vi "CountPulses60.vi"(9 "60bit input":bool[](array[boolean])=[FALSE, FALSE, FALSE, FALSE, FALSE, FALSE, FALSE, FALSE, FALSE, FALSE, FALSE, FALSE, FALSE, FALSE, FALSE, FALSE, FALSE, FALSE, FALSE, FALSE, FALSE, FALSE, FALSE, FALSE, FALSE, FALSE, FALSE, FALSE, FALSE, FALSE, FALSE, FALSE, FALSE, FALSE, FALSE, FALSE, FALSE, FALSE, FALSE, FALSE, FALSE, FALSE, FALSE, FALSE, FALSE, FALSE, FALSE, FALSE, FALSE, FALSE, FALSE, FALSE, FALSE, FALSE, FALSE, FALSE, FALSE, FALSE, FALSE, FALSE], 10 "Previous pulse count":u16, 11 "Last sample":bool) -> (2 "New pulse count":u16, 3 "New last sample":bool)   [LabVIEW 2012]
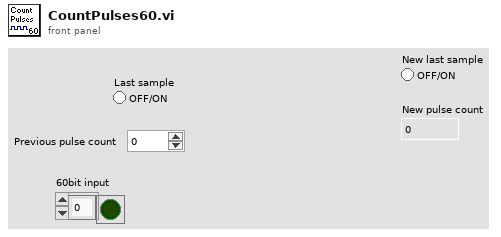
[diagram p1: front panel]
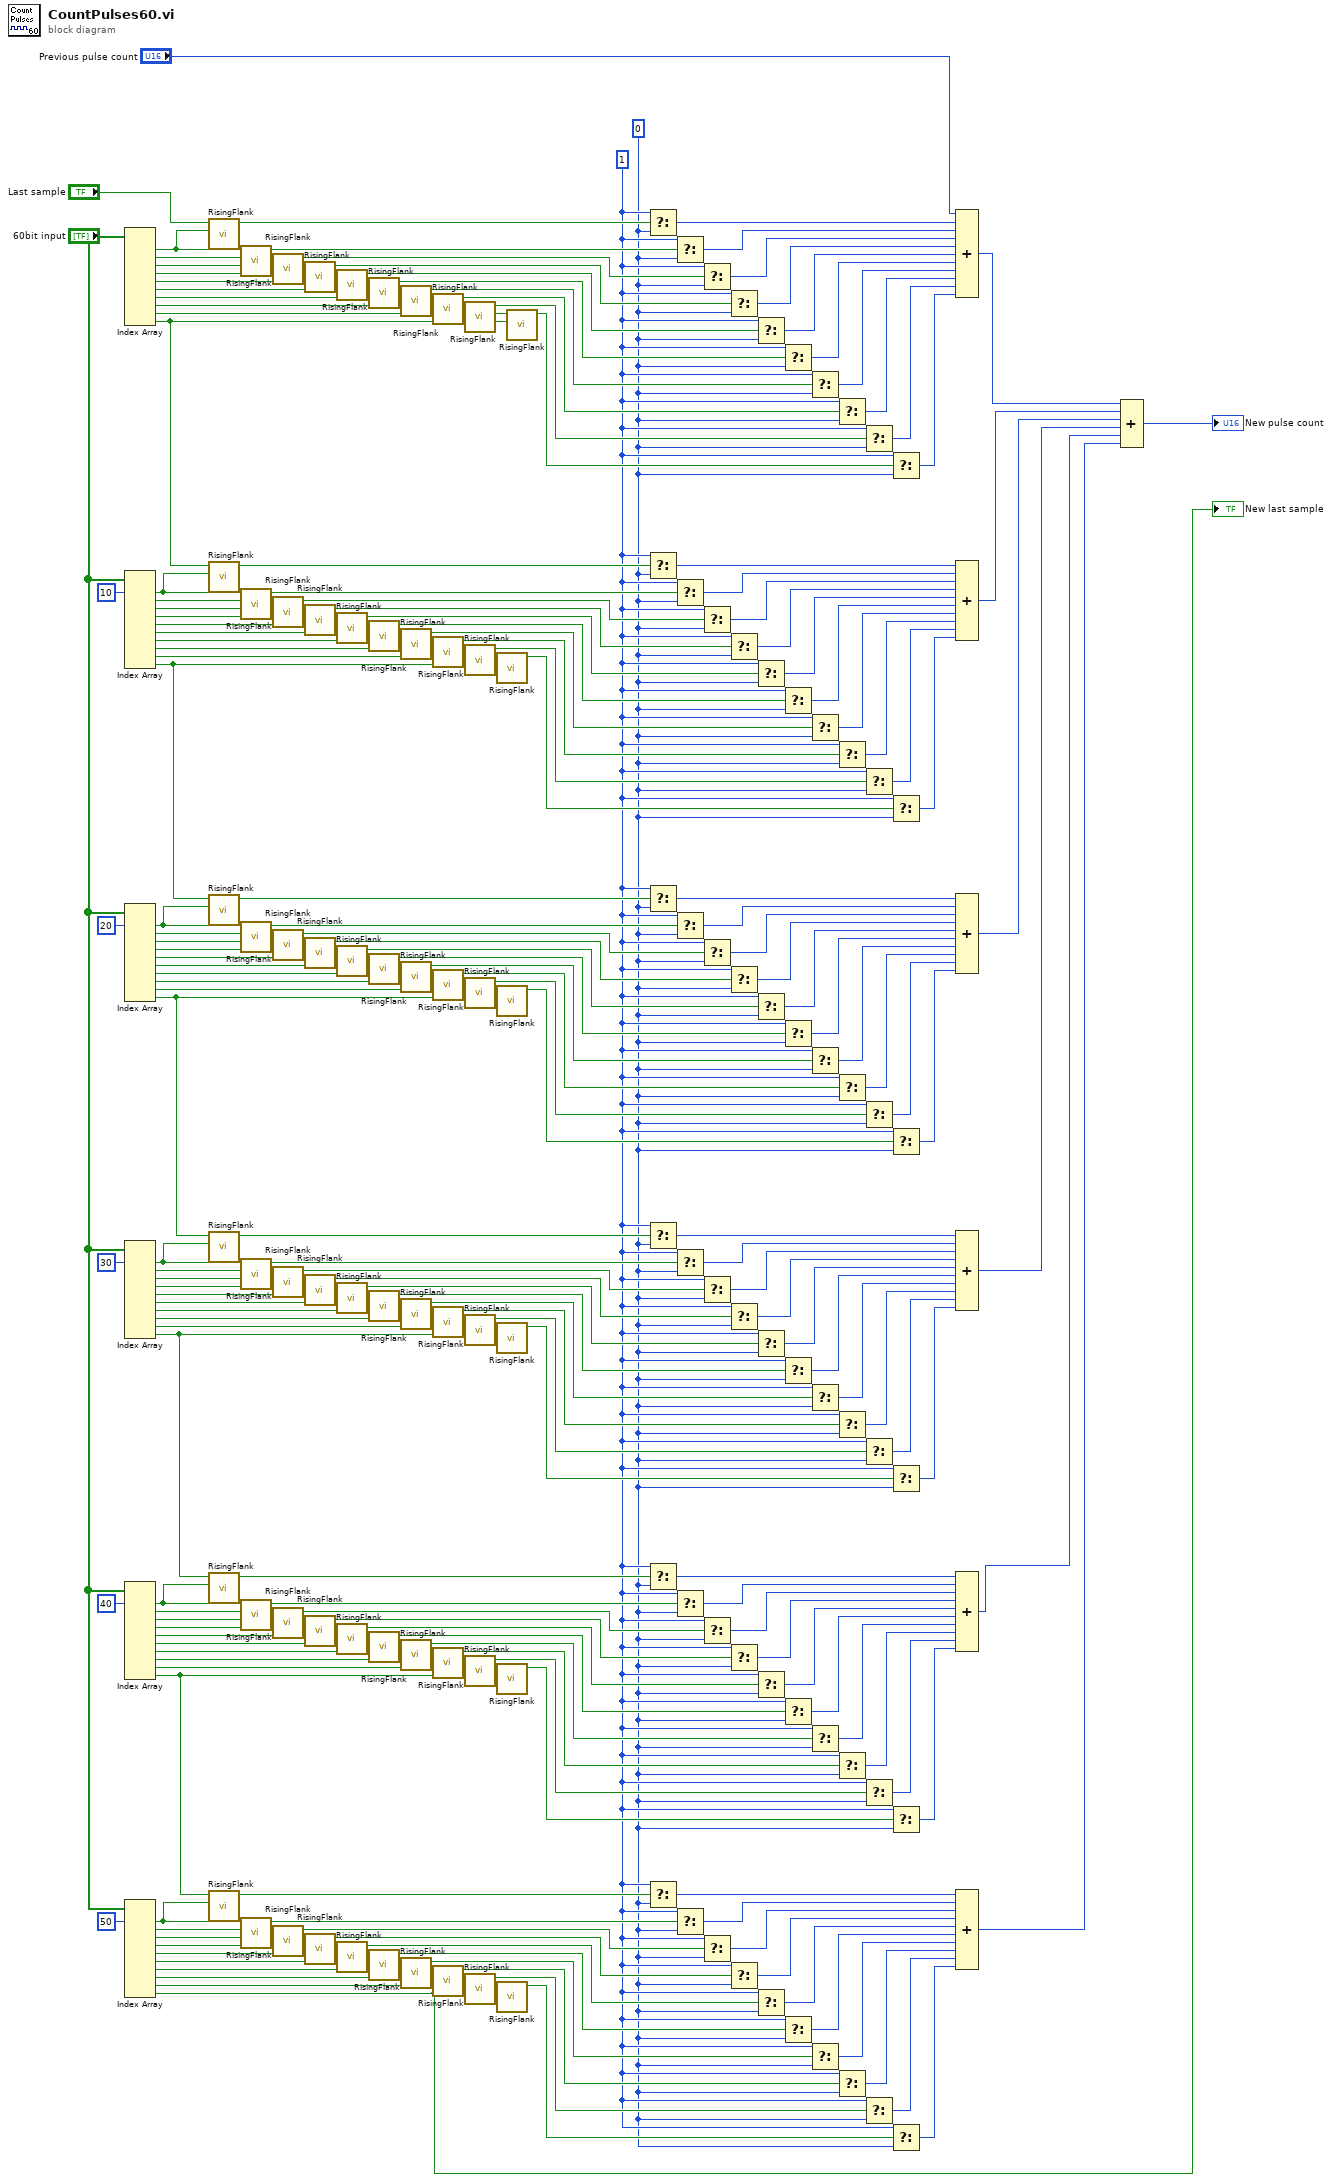
[diagram p0: block diagram]
diagram:
  w11 = u16 1
  w10 = u16 0
  n1 = Index Array(array="60bit input") -> (element #1=w139:bool, element #2=w197:bool, element #3=w196:bool, element #4=w195:bool, element #5=w194:bool, element #6=w193:bool, element #7=w192:bool, element #8=w191:bool, element #9=w190:bool, element #10=w138:bool)  [unwired: 10 in]
  n2 = Index Array(array="60bit input", index #1=10 ("index")) -> (element #1=w137:bool, element #2=w169:bool, element #3=w168:bool, element #4=w167:bool, element #5=w166:bool, element #6=w165:bool, element #7=w164:bool, element #8=w163:bool, element #9=w162:bool, element #10=w106:bool)  [unwired: 9 in]
  n3 = Index Array(array="60bit input", index #1=20 ("index")) -> (element #1=w107:bool, element #2=w136:bool, element #3=w135:bool, element #4=w134:bool, element #5=w133:bool, element #6=w132:bool, element #7=w131:bool, element #8=w130:bool, element #9=w129:bool, element #10=w75:bool)  [unwired: 9 in]
  n4 = Index Array(array="60bit input", index #1=30 ("index")) -> (element #1=w76:bool, element #2=w105:bool, element #3=w104:bool, element #4=w103:bool, element #5=w102:bool, element #6=w101:bool, element #7=w100:bool, element #8=w99:bool, element #9=w98:bool, element #10=w44:bool)  [unwired: 9 in]
  n5 = Index Array(array="60bit input", index #1=40 ("index")) -> (element #1=w45:bool, element #2=w74:bool, element #3=w73:bool, element #4=w72:bool, element #5=w71:bool, element #6=w70:bool, element #7=w69:bool, element #8=w68:bool, element #9=w67:bool, element #10=w12:bool)  [unwired: 9 in]
  n6 = Index Array(array="60bit input", index #1=50 ("index")) -> (element #1=w14:bool, element #2=w43:bool, element #3=w42:bool, element #4=w41:bool, element #5=w40:bool, element #6=w39:bool, element #7=w38:bool, element #8=w37:bool, element #9=w36:bool, element #10=w2:bool)  [unwired: 9 in]
  "New last sample" <- w2
  n7 = call "RisingFlank.vi"("2nd sample"=w139, "1st sample"="Last sample") -> ("Rising flank?"=w189:bool)  [unwired: 7 in]
  n8 = call "RisingFlank.vi"("2nd sample"=w137, "1st sample"=w138) -> ("Rising flank?"=w161:bool)  [unwired: 7 in]
  n9 = call "RisingFlank.vi"("2nd sample"=w107, "1st sample"=w106) -> ("Rising flank?"=w128:bool)  [unwired: 7 in]
  n10 = call "RisingFlank.vi"("2nd sample"=w76, "1st sample"=w75) -> ("Rising flank?"=w97:bool)  [unwired: 7 in]
  n11 = call "RisingFlank.vi"("2nd sample"=w45, "1st sample"=w44) -> ("Rising flank?"=w66:bool)  [unwired: 7 in]
  n12 = call "RisingFlank.vi"("2nd sample"=w14, "1st sample"=w12) -> ("Rising flank?"=w35:bool)  [unwired: 7 in]
  n13 = call "RisingFlank.vi"("2nd sample"=w197, "1st sample"=w139) -> ("Rising flank?"=w188:bool)  [unwired: 7 in]
  n14 = call "RisingFlank.vi"("2nd sample"=w169, "1st sample"=w137) -> ("Rising flank?"=w160:bool)  [unwired: 7 in]
  n15 = call "RisingFlank.vi"("2nd sample"=w136, "1st sample"=w107) -> ("Rising flank?"=w127:bool)  [unwired: 7 in]
  n16 = call "RisingFlank.vi"("2nd sample"=w105, "1st sample"=w76) -> ("Rising flank?"=w96:bool)  [unwired: 7 in]
  n17 = call "RisingFlank.vi"("2nd sample"=w74, "1st sample"=w45) -> ("Rising flank?"=w65:bool)  [unwired: 7 in]
  n18 = call "RisingFlank.vi"("2nd sample"=w43, "1st sample"=w14) -> ("Rising flank?"=w34:bool)  [unwired: 7 in]
  n19 = call "RisingFlank.vi"("2nd sample"=w196, "1st sample"=w197) -> ("Rising flank?"=w187:bool)  [unwired: 7 in]
  n20 = call "RisingFlank.vi"("2nd sample"=w168, "1st sample"=w169) -> ("Rising flank?"=w159:bool)  [unwired: 7 in]
  n21 = call "RisingFlank.vi"("2nd sample"=w135, "1st sample"=w136) -> ("Rising flank?"=w126:bool)  [unwired: 7 in]
  n22 = call "RisingFlank.vi"("2nd sample"=w104, "1st sample"=w105) -> ("Rising flank?"=w95:bool)  [unwired: 7 in]
  n23 = call "RisingFlank.vi"("2nd sample"=w73, "1st sample"=w74) -> ("Rising flank?"=w64:bool)  [unwired: 7 in]
  n24 = call "RisingFlank.vi"("2nd sample"=w42, "1st sample"=w43) -> ("Rising flank?"=w33:bool)  [unwired: 7 in]
  n25 = call "RisingFlank.vi"("2nd sample"=w195, "1st sample"=w196) -> ("Rising flank?"=w186:bool)  [unwired: 7 in]
  n26 = call "RisingFlank.vi"("2nd sample"=w167, "1st sample"=w168) -> ("Rising flank?"=w158:bool)  [unwired: 7 in]
  n27 = call "RisingFlank.vi"("2nd sample"=w134, "1st sample"=w135) -> ("Rising flank?"=w125:bool)  [unwired: 7 in]
  n28 = call "RisingFlank.vi"("2nd sample"=w103, "1st sample"=w104) -> ("Rising flank?"=w94:bool)  [unwired: 7 in]
  n29 = call "RisingFlank.vi"("2nd sample"=w72, "1st sample"=w73) -> ("Rising flank?"=w63:bool)  [unwired: 7 in]
  n30 = call "RisingFlank.vi"("2nd sample"=w41, "1st sample"=w42) -> ("Rising flank?"=w32:bool)  [unwired: 7 in]
  n31 = call "RisingFlank.vi"("2nd sample"=w194, "1st sample"=w195) -> ("Rising flank?"=w185:bool)  [unwired: 7 in]
  n32 = call "RisingFlank.vi"("2nd sample"=w166, "1st sample"=w167) -> ("Rising flank?"=w157:bool)  [unwired: 7 in]
  n33 = call "RisingFlank.vi"("2nd sample"=w133, "1st sample"=w134) -> ("Rising flank?"=w124:bool)  [unwired: 7 in]
  n34 = call "RisingFlank.vi"("2nd sample"=w102, "1st sample"=w103) -> ("Rising flank?"=w93:bool)  [unwired: 7 in]
  n35 = call "RisingFlank.vi"("2nd sample"=w71, "1st sample"=w72) -> ("Rising flank?"=w62:bool)  [unwired: 7 in]
  n36 = call "RisingFlank.vi"("2nd sample"=w40, "1st sample"=w41) -> ("Rising flank?"=w31:bool)  [unwired: 7 in]
  n37 = call "RisingFlank.vi"("2nd sample"=w193, "1st sample"=w194) -> ("Rising flank?"=w184:bool)  [unwired: 7 in]
  n38 = call "RisingFlank.vi"("2nd sample"=w165, "1st sample"=w166) -> ("Rising flank?"=w156:bool)  [unwired: 7 in]
  n39 = call "RisingFlank.vi"("2nd sample"=w132, "1st sample"=w133) -> ("Rising flank?"=w123:bool)  [unwired: 7 in]
  n40 = call "RisingFlank.vi"("2nd sample"=w101, "1st sample"=w102) -> ("Rising flank?"=w92:bool)  [unwired: 7 in]
  n41 = call "RisingFlank.vi"("2nd sample"=w70, "1st sample"=w71) -> ("Rising flank?"=w61:bool)  [unwired: 7 in]
  n42 = call "RisingFlank.vi"("2nd sample"=w39, "1st sample"=w40) -> ("Rising flank?"=w30:bool)  [unwired: 7 in]
  n43 = call "RisingFlank.vi"("2nd sample"=w192, "1st sample"=w193) -> ("Rising flank?"=w183:bool)  [unwired: 7 in]
  n44 = call "RisingFlank.vi"("2nd sample"=w164, "1st sample"=w165) -> ("Rising flank?"=w155:bool)  [unwired: 7 in]
  n45 = call "RisingFlank.vi"("2nd sample"=w131, "1st sample"=w132) -> ("Rising flank?"=w122:bool)  [unwired: 7 in]
  n46 = call "RisingFlank.vi"("2nd sample"=w100, "1st sample"=w101) -> ("Rising flank?"=w91:bool)  [unwired: 7 in]
  n47 = call "RisingFlank.vi"("2nd sample"=w69, "1st sample"=w70) -> ("Rising flank?"=w60:bool)  [unwired: 7 in]
  n48 = call "RisingFlank.vi"("2nd sample"=w38, "1st sample"=w39) -> ("Rising flank?"=w29:bool)  [unwired: 7 in]
  n49 = call "RisingFlank.vi"("2nd sample"=w191, "1st sample"=w192) -> ("Rising flank?"=w182:bool)  [unwired: 7 in]
  n50 = call "RisingFlank.vi"("2nd sample"=w163, "1st sample"=w164) -> ("Rising flank?"=w154:bool)  [unwired: 7 in]
  n51 = call "RisingFlank.vi"("2nd sample"=w130, "1st sample"=w131) -> ("Rising flank?"=w121:bool)  [unwired: 7 in]
  n52 = call "RisingFlank.vi"("2nd sample"=w99, "1st sample"=w100) -> ("Rising flank?"=w90:bool)  [unwired: 7 in]
  n53 = call "RisingFlank.vi"("2nd sample"=w68, "1st sample"=w69) -> ("Rising flank?"=w59:bool)  [unwired: 7 in]
  n54 = call "RisingFlank.vi"("2nd sample"=w37, "1st sample"=w38) -> ("Rising flank?"=w28:bool)  [unwired: 7 in]
  n55 = call "RisingFlank.vi"("2nd sample"=w190, "1st sample"=w191) -> ("Rising flank?"=w181:bool)  [unwired: 7 in]
  n56 = call "RisingFlank.vi"("2nd sample"=w162, "1st sample"=w163) -> ("Rising flank?"=w153:bool)  [unwired: 7 in]
  n57 = call "RisingFlank.vi"("2nd sample"=w129, "1st sample"=w130) -> ("Rising flank?"=w120:bool)  [unwired: 7 in]
  n58 = call "RisingFlank.vi"("2nd sample"=w98, "1st sample"=w99) -> ("Rising flank?"=w89:bool)  [unwired: 7 in]
  n59 = call "RisingFlank.vi"("2nd sample"=w67, "1st sample"=w68) -> ("Rising flank?"=w58:bool)  [unwired: 7 in]
  n60 = call "RisingFlank.vi"("2nd sample"=w36, "1st sample"=w37) -> ("Rising flank?"=w27:bool)  [unwired: 7 in]
  n61 = call "RisingFlank.vi"("2nd sample"=w106, "1st sample"=w162) -> ("Rising flank?"=w152:bool)  [unwired: 7 in]
  n62 = call "RisingFlank.vi"("2nd sample"=w75, "1st sample"=w129) -> ("Rising flank?"=w119:bool)  [unwired: 7 in]
  n63 = call "RisingFlank.vi"("2nd sample"=w44, "1st sample"=w98) -> ("Rising flank?"=w88:bool)  [unwired: 7 in]
  n64 = call "RisingFlank.vi"("2nd sample"=w12, "1st sample"=w67) -> ("Rising flank?"=w57:bool)  [unwired: 7 in]
  n65 = call "RisingFlank.vi"("2nd sample"=w2, "1st sample"=w36) -> ("Rising flank?"=w26:bool)  [unwired: 7 in]
  n66 = call "RisingFlank.vi"("2nd sample"=w138, "1st sample"=w190) -> ("Rising flank?"=w180:bool)  [unwired: 7 in]
  n67 = Select(t=w11, s=w189, f=w10) -> (s? t:f=w179:u16)
  n68 = Select(t=w11, s=w161, f=w10) -> (s? t:f=w151:u16)
  n69 = Select(t=w11, s=w128, f=w10) -> (s? t:f=w118:u16)
  n70 = Select(t=w11, s=w97, f=w10) -> (s? t:f=w87:u16)
  n71 = Select(t=w11, s=w66, f=w10) -> (s? t:f=w56:u16)
  n72 = Select(t=w11, s=w35, f=w10) -> (s? t:f=w25:u16)
  n73 = Select(t=w11, s=w188, f=w10) -> (s? t:f=w178:u16)
  n74 = Select(t=w11, s=w160, f=w10) -> (s? t:f=w150:u16)
  n75 = Select(t=w11, s=w127, f=w10) -> (s? t:f=w117:u16)
  n76 = Select(t=w11, s=w96, f=w10) -> (s? t:f=w86:u16)
  n77 = Select(t=w11, s=w65, f=w10) -> (s? t:f=w55:u16)
  n78 = Select(t=w11, s=w34, f=w10) -> (s? t:f=w24:u16)
  n79 = Select(t=w11, s=w187, f=w10) -> (s? t:f=w177:u16)
  n80 = Select(t=w11, s=w159, f=w10) -> (s? t:f=w149:u16)
  n81 = Select(t=w11, s=w126, f=w10) -> (s? t:f=w116:u16)
  n82 = Select(t=w11, s=w95, f=w10) -> (s? t:f=w85:u16)
  n83 = Select(t=w11, s=w64, f=w10) -> (s? t:f=w54:u16)
  n84 = Select(t=w11, s=w33, f=w10) -> (s? t:f=w23:u16)
  n85 = Select(t=w11, s=w186, f=w10) -> (s? t:f=w176:u16)
  n86 = Select(t=w11, s=w158, f=w10) -> (s? t:f=w148:u16)
  n87 = Select(t=w11, s=w125, f=w10) -> (s? t:f=w115:u16)
  n88 = Select(t=w11, s=w94, f=w10) -> (s? t:f=w84:u16)
  n89 = Select(t=w11, s=w63, f=w10) -> (s? t:f=w53:u16)
  n90 = Select(t=w11, s=w32, f=w10) -> (s? t:f=w22:u16)
  n91 = Select(t=w11, s=w185, f=w10) -> (s? t:f=w175:u16)
  n92 = Select(t=w11, s=w157, f=w10) -> (s? t:f=w147:u16)
  n93 = Select(t=w11, s=w124, f=w10) -> (s? t:f=w114:u16)
  n94 = Select(t=w11, s=w93, f=w10) -> (s? t:f=w83:u16)
  n95 = Select(t=w11, s=w62, f=w10) -> (s? t:f=w52:u16)
  n96 = Select(t=w11, s=w31, f=w10) -> (s? t:f=w21:u16)
  n97 = Select(t=w11, s=w184, f=w10) -> (s? t:f=w174:u16)
  n98 = Select(t=w11, s=w156, f=w10) -> (s? t:f=w146:u16)
  n99 = Select(t=w11, s=w123, f=w10) -> (s? t:f=w113:u16)
  n100 = Select(t=w11, s=w92, f=w10) -> (s? t:f=w82:u16)
  n101 = Select(t=w11, s=w61, f=w10) -> (s? t:f=w51:u16)
  n102 = Select(t=w11, s=w30, f=w10) -> (s? t:f=w20:u16)
  n103 = Select(t=w11, s=w183, f=w10) -> (s? t:f=w173:u16)
  n104 = Select(t=w11, s=w155, f=w10) -> (s? t:f=w145:u16)
  n105 = Select(t=w11, s=w122, f=w10) -> (s? t:f=w112:u16)
  n106 = Select(t=w11, s=w91, f=w10) -> (s? t:f=w81:u16)
  n107 = Select(t=w11, s=w60, f=w10) -> (s? t:f=w50:u16)
  n108 = Select(t=w11, s=w29, f=w10) -> (s? t:f=w19:u16)
  n109 = Select(t=w11, s=w182, f=w10) -> (s? t:f=w172:u16)
  n110 = Select(t=w11, s=w154, f=w10) -> (s? t:f=w144:u16)
  n111 = Select(t=w11, s=w121, f=w10) -> (s? t:f=w111:u16)
  n112 = Select(t=w11, s=w90, f=w10) -> (s? t:f=w80:u16)
  n113 = Select(t=w11, s=w59, f=w10) -> (s? t:f=w49:u16)
  n114 = Select(t=w11, s=w28, f=w10) -> (s? t:f=w18:u16)
  n115 = Select(t=w11, s=w181, f=w10) -> (s? t:f=w171:u16)
  n116 = Select(t=w11, s=w153, f=w10) -> (s? t:f=w143:u16)
  n117 = Select(t=w11, s=w120, f=w10) -> (s? t:f=w110:u16)
  n118 = Select(t=w11, s=w89, f=w10) -> (s? t:f=w79:u16)
  n119 = Select(t=w11, s=w58, f=w10) -> (s? t:f=w48:u16)
  n120 = Select(t=w11, s=w27, f=w10) -> (s? t:f=w17:u16)
  n121 = Select(t=w11, s=w180, f=w10) -> (s? t:f=w170:u16)
  n122 = Select(t=w11, s=w152, f=w10) -> (s? t:f=w142:u16)
  n123 = Select(t=w11, s=w119, f=w10) -> (s? t:f=w109:u16)
  n124 = Select(t=w11, s=w88, f=w10) -> (s? t:f=w78:u16)
  n125 = Select(t=w11, s=w57, f=w10) -> (s? t:f=w47:u16)
  n126 = Select(t=w11, s=w26, f=w10) -> (s? t:f=w16:u16)
  n127 = Compound Arithmetic op=ADD("Previous pulse count", w179, w178, w177, w176, w175, w174, w173, w172, w171, w170) -> (w9:u16)
  n128 = Compound Arithmetic op=ADD(w151, w150, w149, w148, w147, w146, w145, w144, w143, w142) -> (w7:u16)
  n129 = Compound Arithmetic op=ADD(w118, w117, w116, w115, w114, w113, w112, w111, w110, w109) -> (w6:u16)
  n130 = Compound Arithmetic op=ADD(w87, w86, w85, w84, w83, w82, w81, w80, w79, w78) -> (w5:u16)
  n131 = Compound Arithmetic op=ADD(w56, w55, w54, w53, w52, w51, w50, w49, w48, w47) -> (w4:u16)
  n132 = Compound Arithmetic op=ADD(w25, w24, w23, w22, w21, w20, w19, w18, w17, w16) -> (w3:u16)
  n133 = Compound Arithmetic op=ADD(w9, w7, w6, w5, w4, w3) -> (→"New pulse count":u16)
